vi "R45_2-RT.vi"() -> ()   [LabVIEW 2016]
uses:
  Faraday cup states.ctl
  Aperture states.ctl
  GV states.ctl
  <vilib>/Platform/TimedLoop/XDataNode/timing_clust.ctl
  <vilib>/Platform/TimedLoop/XDataNode/nitl_modes.ctl
  <vilib>/Platform/TimedLoop/XDataNode/wakeup.ctl
  Glassman Control.ctl
  GP307 cluster.ctl
  <vilib>/FPGAPlugInAG/cRIO-9074/niLvFpga_Open_cRIO-9074.vi
  <vilib>/Utility/error.llb/Error Cluster From Error Code.vi
  <vilib>/rvi/errors/niLvFpgaAdjustHostInterfaceError.vi
  <vilib>/functionblocks/Control/PID/PID.vi
  <vilib>/rvi/interface/nirviOpenFPGA/nirviOpenFPGA.xnode
  Slow-Switching-Control/FPGA Bitfiles/Controlsoftware2_FPGATarget8_R45-2-FPGA_XDn2JZv1h+E.lvbitx
  R45_2-FPGA.vi
  <vilib>/Platform/TimedLoop/XDataNode/XDataNode.xnode
  <vilib>/rvi/interface/nirviReadWriteControl/nirviReadWriteControl.xnode
  <vilib>/functionblocks/FB Core/FB Core.xnode
  Gate Valve Readback.ctl
  Aperture Readback.ctl
  Faraday Cup Readback.ctl
  Glassman Readback.ctl
  <vilib>/Platform/TimedLoop/XDataNode/XDNodeRunTimeDep.lvlib
  <vilib>/functionblocks/NI_FunctionBlock Libraries.lvlib
  NiFpgaLv.dll
panel:
  out "Error Reporter":errorcluster
  in  "Tab Control":T1(tab)
  out "HV readback loop error":errorcluster
  out "R45 ExB 1 HV Enable":bool
  out "R45 ExB 1 voltage set":dbl
  out "HV control loop error":errorcluster
  out "ExB 1- I read":dbl
  out "ExB 1- V read":dbl
  out "ExB 2+ I read":dbl
  out "ExB 2+ V read":dbl
  out "ExB 2- I read":dbl
  out "ExB 2- V read":dbl
  out "X-steerer Mag I read":dbl
  out "X-steerer Mag V read":dbl
  out "R45 ExB 2 HV Enable":bool
  out "R45 ExB 2 voltage set":dbl
  out "X-Steerer Magnet current set":dbl
  out "ExB 1+ I read":dbl
  out "ExB 1+ V read":dbl
  out "GRM magnet current set":dbl
  out "GFM read string":string
  in  "proportional gain (Kc) - GFM":dbl=1.0
  in  "integral time (Ti, min) - GFM":dbl=0.01
  in  "derivative time (Td, min) - GFM":dbl
  in  "output high - GFM":dbl=205.0
  in  "output low - GFM":dbl
  out "GFM field read":u8[](array[numeric])
  out "GFM field":dbl format="%#_8f"
  out "GFM loop error":errorcluster
  out "ExB 2 PS loop error":errorcluster
  out "ExB 1 PS loop error":errorcluster
  out "GFM command":u8[](array[numeric])
  out "R45 ExB 2 command string":string
  out "R45 ExB 2 command array":u8[](array[numeric])
  out "ExB #2 magnet current set":dbl
  out "GFM command string":string
  out "GFM field set":dbl
  out "ExB #1 magnet current set":dbl
  out "R45 ExB 1 command string":string
  out "R45 ExB 1 command array":u8[](array[numeric])
  out "Vacuum readback error":errorcluster
  out "Ion Gauge 3-2":u8[](array[numeric])
  out "Convectron gauge 3-2":u8[](array[numeric])
  out "Ion gauge 2-2":u8[](array[numeric])
  out "Ion gauge 2-1":u8[](array[numeric])
  out "Convectron 3-1":u8[](array[numeric])
  out "Ion gauge 3-1":u8[](array[numeric])
  out "Convectron 2-2":u8[](array[numeric])
  out "Convectron 2-1":u8[](array[numeric])
  out "Ion Gauge 4-1":u8[](array[numeric])
  out "Convectron Gauge 4-1":u8[](array[numeric])
  out "Ion Gauge 4-2":u8[](array[numeric])
  out "Convectron Gauge 4-2":u8[](array[numeric])
  out "R45 Quad  vac gauge cluster":T2
  out "R45 Detector vac gauge cluster":T2
  out "R45 ExB Slot vac gauge cluster":T2
  out "Vac cluster 2 Ion Guage Interlock":bool
  out "Vac cluster 3 Ion Guage Interlock":bool
  out "Vac cluster 4 Ion Guage Interlock":bool
  out "Interlock readbacks Loop error":errorcluster
  out "Vac cluster 1 Gauge Interlock":bool
  out "Vac cluster 1 Interlock bypass":bool
  out "Switch Object Vac Interlock":bool
  out "Switch Object Interlock Bypass":bool
  out "Vac cluster 2 Interlock bypass":bool
  out "Vac cluster 4 Interlock bypass":bool
  out "Vac cluster 3 Interlock bypass":bool
  out "Turbo 2 GV Status":T3
  out "Turbo 1 GV Status":T3
  out "Beamline GV 3 Status":T3
  out "Beamline GV 2 Status":T3
  out "R45 Switching Mag GV Status":T3
  out "Turbo 3 GV Status":T3
  out "Detector FC status":T4
  out "Detector Aperture status":T5
  out "Detector Aperture Position":cluster{"IN sensor":bool, "OUT sensor":bool}
  out "Turbo 3 GV Status":T6
  out "Turbo 2 GV Status":T6
  out "Beamline GV 3 Status":T6
  out "Turbo 1 GV Status":T6
  out "R45 Switching Mag GV Status":T6
  out "ExB Slot Aperture Position":cluster{"IN sensor":bool, "OUT sensor":bool}
  out "Detector FC Position":cluster{"IN sensor":bool, "OUT sensor":bool}
  out "Beamline GV 2 Status":T6
  out "ExB Slot Aperture Status":T5
  out "Actuator loop error":errorcluster
  out "R45 Detector FC insert":bool
  out "R45 Detector Aperture insert":bool
  out "R45 ExB Slot Aperture insert":bool
  out "R45 Turbo 3 GV":bool
  out "R45 Turbo 2 GV":bool
  out "R45 Switching Magnet GV":bool
  out "R45 Turbo 1 GV":bool
  out "R45 Beamline GV 3":bool
  out "R45 Beamline GV 2":bool
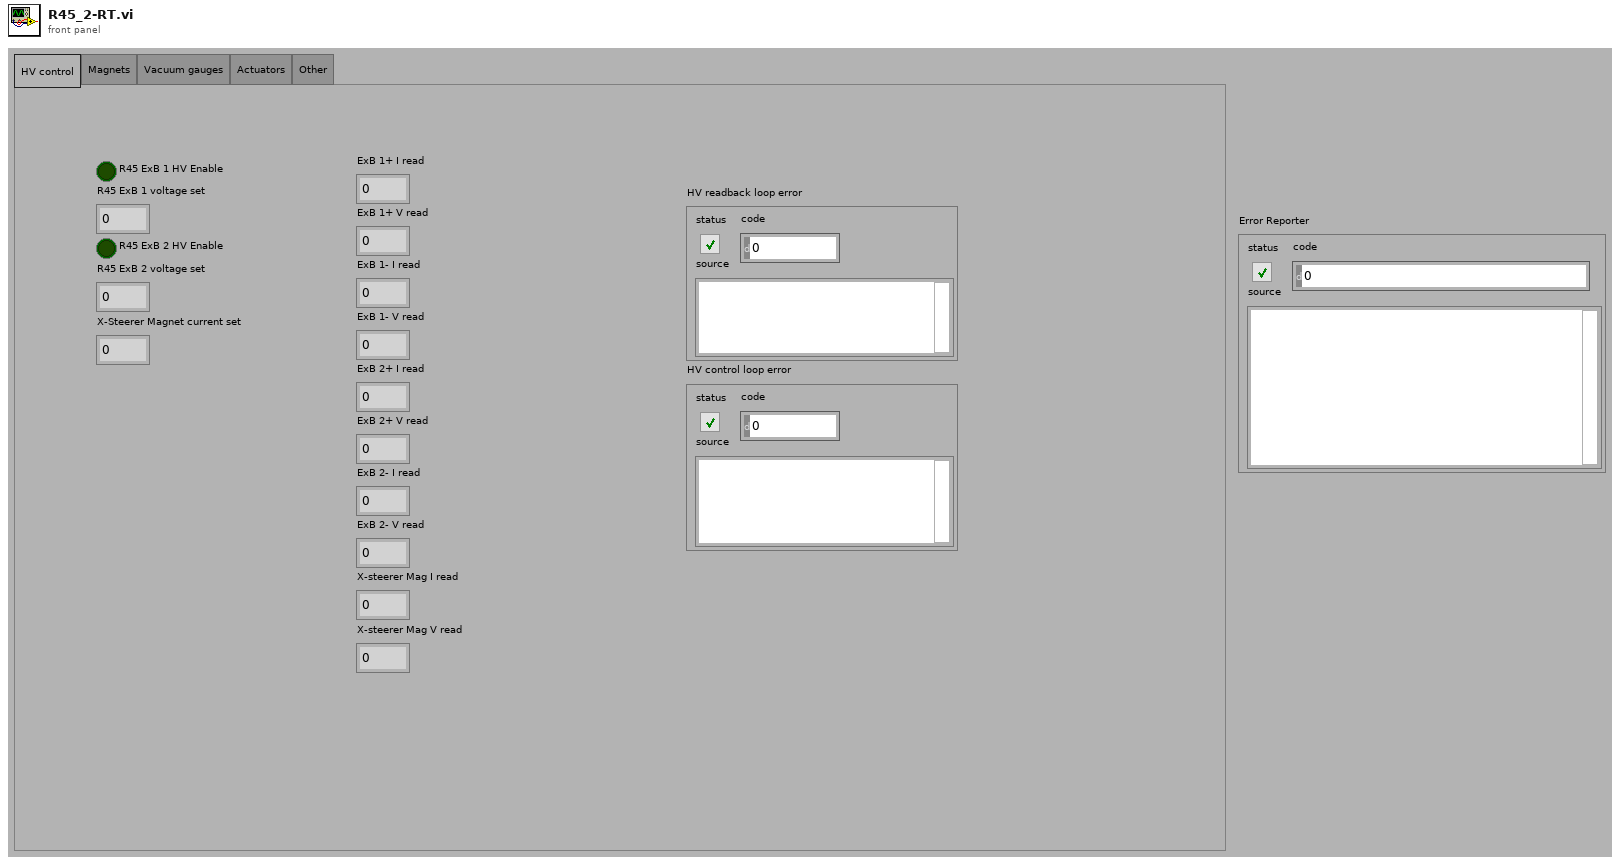
[diagram p1: front panel]
types:
  T1 = enum32{"HV control", "Magnets", "Vacuum gauges", "Actuators", "Other"}
  T2 = cluster{"Ion gauge 1":string, "Convectron  Gauge 1 ":string, "Ion Gauge 2":string, "Convectrom Gauge 2":string}
  T3 = typedef "GV states.ctl" = enum16{"status unclear", "closed", "open"}
  T4 = typedef "Faraday cup states.ctl" = enum16{"FC status unclear", "FC in", "FC out"}
  T5 = typedef "Aperture states.ctl" = enum16{"Aperture status unclear", "Aperture in", "Aperture out"}
  T6 = cluster{"OPEN sensor":bool, "Closed sensor":bool}
  T7 = typedef "XDNodeRunTimeDep.lvlib/timing_clust.ctl" = cluster{"Expected End [f-1]":u64, "Actual End [f-1]":u64, "Finished Late? [f-1]":bool, "Expected End [i-1]":u64, "Actual End [i-1]":u64, "Finished Late? [i-1]":bool, "Expected Start [i]":u64, "Actual Start [i]":u64, "Expected Start [f]":u64, "Actual Start [f]":u64, "Source Name":string, "Structure Name":string, "Period":i64, "Deadline":i64, "Offset":i64, "Start":i64, "Priority":i32, "Timeout":i32, "Mode":T8, "Wakeup Reason":T9, "Error":errorcluster, "Source Type":string, "Secondary Source Type":string, "Global End Time":u64, "Global Start Time":u64, "Frame Duration":u64, "Iteration Duration":u64, "Assigned CPU":i32, "I/O Scan Engine Mode":u32}
  T8 = typedef "XDNodeRunTimeDep.lvlib/nitl_modes.ctl" = enum32{"No Change", "Process missed periods, maintain original phase", "Discard missed periods, maintain original phase", "Process missed periods, ignore original phase", "Discard missed periods, ignore original phase"}
  T9 = typedef "XDNodeRunTimeDep.lvlib/wakeup.ctl" = enum32{"Normal", "Aborted", "Asynchronous wakeup", "Timing source error", "Timed loop error", "Timeout"}
  T10 = typedef "GP307 cluster.ctl" = cluster{"Ion gauge 1":string, "Convectron  Gauge 1 ":string, "Ion Gauge 2":string, "Convectrom Gauge 2":string}
  T11 = typedef "Glassman Control.ctl" = cluster{"V-program":fxp<+/-,20,5>, "HV Enable":bool}
  T12 = typedef "Gate Valve Readback.ctl" = cluster{"OPEN sensor":bool, "Closed sensor":bool}
  T13 = typedef "Aperture Readback.ctl" = cluster{"IN sensor":bool, "OUT sensor":bool}
  T14 = typedef "Faraday Cup Readback.ctl" = cluster{"IN sensor":bool, "OUT sensor":bool}
  T15 = typedef "Glassman Readback.ctl" = cluster{"I-monitor":fxp<+/-,26,5>, "V-monitor":fxp<+/-,26,7>}
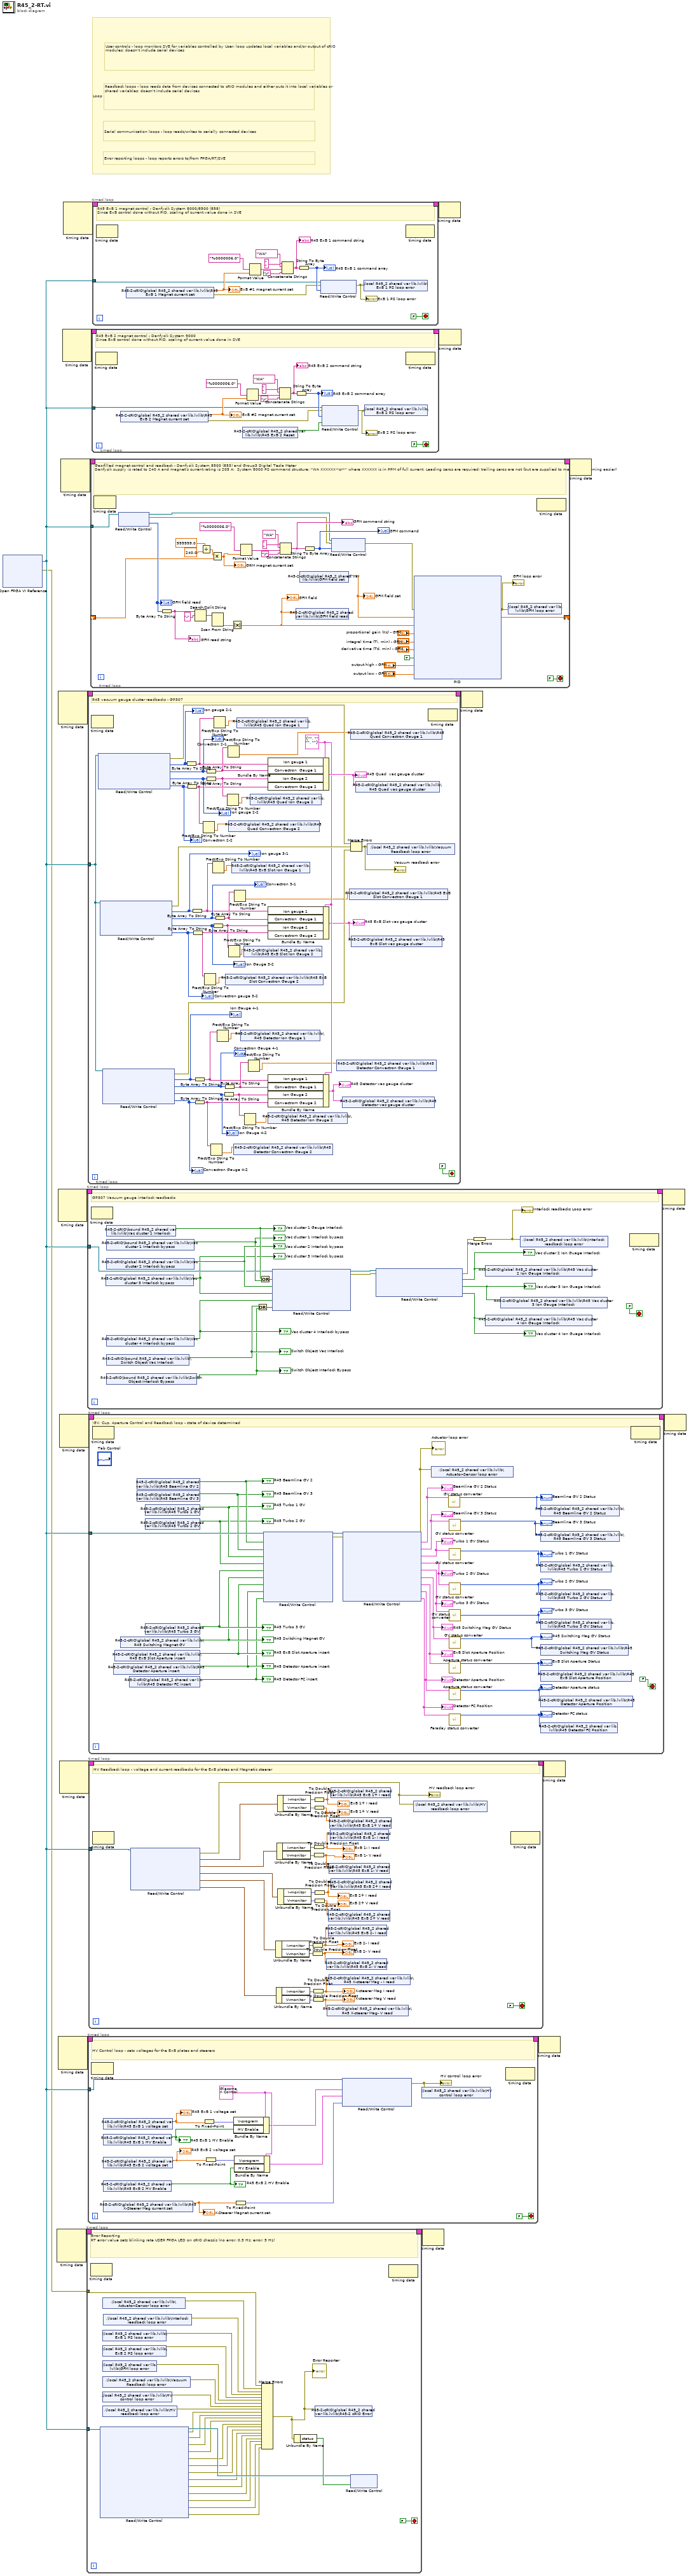
[diagram p0: block diagram]
diagram:
  # "Error reporting loops - loop reports errors to/from FPGA/RT/SVE"
  # "Serial communication loops - loop reads/writes to serially connected devices"
  # "Readback loops - loop reads data from devices connected to cRIO modules and either puts it into local variables or shared variables; doesn't include serial devices"
  # "User controls - loop monitors SVE for variables controlled by User; loop updates local variables and/or output of cRIO modules; doesn't include serial devices"
  # "Loop legend - loops are color coded by responsibility"
  n1 = xnode "Open FPGA VI Reference"() -> ("FPGA VI Reference Out"=w2:refnum<k20>, "error out"=w1:errorcluster)  [unwired: 2 in]
  n2 = node-c288() -> (w8:T7)  [unwired: 4 in]
  n3 = node-c288() -> (w16:T7)  [unwired: 4 in]
  n4 = node-c288() -> (w18:T7)  [unwired: 4 in]
  n5 = node-c288() -> (w6:T7)  [unwired: 4 in]
  n6 = node-c288() -> (w14:T7)  [unwired: 4 in]
  n7 = node-c288() -> (w4:T7)  [unwired: 4 in]
  n8 = node-c288() -> (w20:T7)  [unwired: 4 in]
  n9 = node-c288() -> (w12:T7)  [unwired: 4 in]
  n10 = node-c288() -> (w10:T7)  [unwired: 4 in]
  n11 = timed-loop {
    timing: w8 -> [_]
    timing-out: [_] -> w7
    tunnel: w2 -> [w39]
    tunnel: w1 -> [w23]
    stop <- FALSE stop-if-true
    # "Error Reporting\nRT error value sets blinking rate USER FPGA LED on cRIO chassis (no error: 0.5 Hz; error: 5 Hz)"
    n12 = node-c288() -> ()  [unwired: 1 in, 1 out]
    n13 = xnode "Read/Write Control"("FPGA VI Reference In"=w39) -> ("FPGA VI Reference Out"=w38:refnum<k20>, "error out"=w37:errorcluster, "ExB 1 PS error"=w36:errorcluster, "ExB 2 PS error"=w35:errorcluster, "GFM ps error"=w34:errorcluster, "GFM Hall Probe error"=w33:errorcluster, "HV Readback Loop"=w32:errorcluster, "HV Control Loop error"=w31:errorcluster, "Vacuum Gauge 2 error"=w30:errorcluster, "Vacuum Gauge 3 error"=w29:errorcluster, "Vacuum Gauge 4 error"=w28:errorcluster, "Vac and GV  interlock error"=w24:errorcluster, "Position-Status Sensor error"=w25:errorcluster, "Cup-Aperture Control Loop Error"=w26:errorcluster)  [unwired: 1 in]
    n14 = shared-variable ".\\local R45_2 shared var lib.lvlib\\Actuator-Sensor loop error"() -> (w21:errorcluster)  [unwired: 1 in, 1 out]
    n15 = shared-variable ".\\local R45_2 shared var lib.lvlib\\ExB 1 PS loop error"() -> (w45:errorcluster)  [unwired: 1 in, 1 out]
    n16 = shared-variable ".\\local R45_2 shared var lib.lvlib\\ExB 2 PS loop error"() -> (w44:errorcluster)  [unwired: 1 in, 1 out]
    n17 = shared-variable ".\\local R45_2 shared var lib.lvlib\\GFM loop error"() -> (w43:errorcluster)  [unwired: 1 in, 1 out]
    n18 = shared-variable ".\\local R45_2 shared var lib.lvlib\\Vacuum Readback loop error"() -> (w42:errorcluster)  [unwired: 1 in, 1 out]
    n19 = shared-variable ".\\local R45_2 shared var lib.lvlib\\HV control loop error"() -> (w41:errorcluster)  [unwired: 1 in, 1 out]
    n20 = shared-variable ".\\local R45_2 shared var lib.lvlib\\HV readback loop error"() -> (w40:errorcluster)  [unwired: 1 in, 1 out]
    n21 = shared-variable ".\\local R45_2 shared var lib.lvlib\\Interlock readback loop error"() -> (w22:errorcluster)  [unwired: 1 in, 1 out]
    n22 = Merge Errors(w23, w21, w22, w45, w44, w43, w42, w41, w40, w37, w36, w35, w34, w33, w32, w31, w30, w29, w28, w24, w25, w26) -> (w47:errorcluster)
    "Error Reporter" <- w47
    n23 = Unbundle By Name(w47) -> ("status"=w46:bool)
    n24 = shared-variable "R45-2-cRIO\\global R45_2 shared var lib.lvlib\\R45-2 cRIO Error"(w47) -> ()  [unwired: 1 in, 1 out]
    n25 = xnode "Read/Write Control"("FPGA VI Reference In"=w38, "RT error"=w46) -> ()  [unwired: 1 in, 2 out]
    n26 = node-c288() -> ()  [unwired: 1 in, 1 out]
  }
  n27 = timed-loop {
    tunnel: w2 -> [w55]
    timing: w16 -> [_]
    timing-out: [_] -> w15
    stop <- FALSE stop-if-true
    # "GP307 Vacuum gauge interlock readbacks"
    n28 = node-c288() -> ()  [unwired: 1 in, 1 out]
    n29 = shared-variable "R45-2-cRIO\\global R45_2 shared var lib.lvlib\\Vac cluster 3 Interlock bypass"() -> (w50:bool)  [unwired: 1 in, 1 out]
    "Vac cluster 3 Interlock bypass" <- w50
    n30 = shared-variable "R45-2-cRIO\\bound R45_2 shared var lib.lvlib\\Vac cluster 1 Interlock"() -> (w59:bool)  [unwired: 1 in, 1 out]
    "Vac cluster 1 Gauge Interlock" <- w59
    n31 = shared-variable "R45-2-cRIO\\bound R45_2 shared var lib.lvlib\\Vac cluster 1 Interlock bypass"() -> (w51:bool)  [unwired: 1 in, 1 out]
    "Vac cluster 1 Interlock bypass" <- w51
    n32 = shared-variable "R45-2-cRIO\\global R45_2 shared var lib.lvlib\\Vac cluster 2 Interlock bypass"() -> (w56:bool)  [unwired: 1 in, 1 out]
    "Vac cluster 2 Interlock bypass" <- w56
    n33 = shared-variable "R45-2-cRIO\\global R45_2 shared var lib.lvlib\\Vac cluster 4 Interlock bypass"() -> (w57:bool)  [unwired: 1 in, 1 out]
    "Vac cluster 4 Interlock bypass" <- w57
    n34 = shared-variable "R45-2-cRIO\\bound R45_2 shared var lib.lvlib\\Switch Object Vac Interlock"() -> (w58:bool)  [unwired: 1 in, 1 out]
    "Switch Object Vac Interlock" <- w58
    n35 = shared-variable "R45-2-cRIO\\bound R45_2 shared var lib.lvlib\\Switch Object Interlock Bypass"() -> (w53:bool)  [unwired: 1 in, 1 out]
    "Switch Object Interlock Bypass" <- w53
    n36 = Or(x=w58, y=w53) -> (x .or. y?=w54:bool)
    n37 = Or(x=w59, y=w51) -> (x .or. y?=w52:bool)
    n38 = xnode "Read/Write Control"("FPGA VI Reference In"=w55, "Vac cluster 1 Gauge Interlock"=w52, "Vac cluster 2 Interlock bypass"=w56, "Vac cluster 3 Interlock bypass"=w50, "Vac cluster 4 Interlock bypass"=w57, "Switch Object Interlock"=w54) -> ("FPGA VI Reference Out"=w61:refnum<k20>, "error out"=w60:errorcluster)  [unwired: 1 in]
    n39 = xnode "Read/Write Control"("FPGA VI Reference In"=w61, "error in"=w60) -> ("error out"=w63:errorcluster, "Vac cluster 2 Ion Gauge Interlock"=w64:bool, "Vac cluster 3 Ion Gauge Interlock"=w66:bool, "Vac cluster 4 Ion Gauge Interlock"=w65:bool)  [unwired: 1 out]
    "Vac cluster 2 Ion Guage Interlock" <- w64
    "Vac cluster 3 Ion Guage Interlock" <- w66
    "Vac cluster 4 Ion Guage Interlock" <- w65
    n40 = Merge Errors(w63) -> (w62:errorcluster)
    "Interlock readbacks Loop error" <- w62
    n41 = shared-variable "R45-2-cRIO\\global R45_2 shared var lib.lvlib\\R45 Vac cluster 2 Ion Gauge Interlock"(w64) -> ()  [unwired: 1 in, 1 out]
    n42 = shared-variable "R45-2-cRIO\\global R45_2 shared var lib.lvlib\\R45 Vac cluster 4 Ion Gauge Interlock"(w65) -> ()  [unwired: 1 in, 1 out]
    n43 = shared-variable "R45-2-cRIO\\global R45_2 shared var lib.lvlib\\R45 Vac cluster 3 Ion Gauge Interlock"(w66) -> ()  [unwired: 1 in, 1 out]
    n44 = shared-variable ".\\local R45_2 shared var lib.lvlib\\Interlock readback loop error"(w62) -> ()  [unwired: 1 in, 1 out]
    n45 = node-c288() -> ()  [unwired: 1 in, 1 out]
  }
  n46 = timed-loop {
    tunnel: w2 -> [w93]
    timing: w18 -> [_]
    timing-out: [_] -> w17
    stop <- FALSE stop-if-true
    w104 = T10 {"Ion gauge 1"="", "Convectron  Gauge 1 "="", "Ion Gauge 2"="", "Convectrom Gauge 2"=""} ("Ion gauge cluster control")
    # "R45 vacuum gauge cluster readbacks - GP307"
    n47 = node-c288() -> ()  [unwired: 1 in, 1 out]
    n48 = xnode "Read/Write Control"("FPGA VI Reference In"=w93) -> ("error out"=w83:errorcluster, "Vac Cluster 2 Ion Gauge 1"=w92:u8[], "Vac Cluster 2 Convectron 1"=w91:u8[], "Vac Cluster 2 Ion Gauge 2"=w90:u8[], "Vac Cluster 2 Convectron 2"=w89:u8[])  [unwired: 1 in, 1 out]
    "Ion gauge 2-1" <- w92
    "Convectron 2-1" <- w91
    "Ion gauge 2-2" <- w90
    "Convectron 2-2" <- w89
    n49 = xnode "Read/Write Control"("FPGA VI Reference In"=w93) -> ("error out"=w115:errorcluster, "Vac Cluster 3 Ion Gauge 1"=w113:u8[], "Vac Cluster 3 Convectron 1"=w112:u8[], "Vac Cluster 3 Convectron 2"=w110:u8[], "Vac Cluster 3 Convectron 2"=w111:u8[])  [unwired: 1 in, 1 out]
    "Ion gauge 3-1" <- w113
    "Convectron 3-1" <- w112
    "Convectron gauge 3-2" <- w111
    "Ion Gauge 3-2" <- w110
    n50 = xnode "Read/Write Control"("FPGA VI Reference In"=w93) -> ("error out"=w82:errorcluster, "Vac Cluster 4 Ion Gauge 1"=w96:u8[], "Vac Cluster 4 Convectron 1"=w98:u8[], "Vac Cluster 4 Ion Gauge 2"=w99:u8[], "Vac Cluster 4 Convectron 2"=w97:u8[])  [unwired: 1 in, 1 out]
    "Ion Gauge 4-1" <- w96
    "Convectron Gauge 4-1" <- w98
    "Ion Gauge 4-2" <- w99
    "Convectron Gauge 4-2" <- w97
    n51 = Byte Array To String(unsigned byte array=w92) -> (string=w108:string)
    n52 = Byte Array To String(unsigned byte array=w89) -> (string=w86:string)
    n53 = Byte Array To String(unsigned byte array=w113) -> (string=w107:string)
    n54 = Byte Array To String(unsigned byte array=w111) -> (string=w88:string)
    n55 = Byte Array To String(unsigned byte array=w96) -> (string=w100:string)
    n56 = Byte Array To String(unsigned byte array=w97) -> (string=w94:string)
    n57 = Fract/Exp String To Number(string=w86) -> (number=w71:dbl)  [unwired: 3 in, 1 out]
    n58 = Fract/Exp String To Number(string=w88) -> (number=w75:dbl)  [unwired: 3 in, 1 out]
    n59 = Byte Array To String(unsigned byte array=w91) -> (string=w105:string)
    n60 = Byte Array To String(unsigned byte array=w90) -> (string=w85:string)
    n61 = Fract/Exp String To Number(string=w94) -> (number=w78:dbl)  [unwired: 3 in, 1 out]
    n62 = Fract/Exp String To Number(string=w107) -> (number=w77:dbl)  [unwired: 3 in, 1 out]
    n63 = Byte Array To String(unsigned byte array=w110) -> (string=w87:string)
    n64 = Fract/Exp String To Number(string=w108) -> (number=w73:dbl)  [unwired: 3 in, 1 out]
    n65 = Byte Array To String(unsigned byte array=w112) -> (string=w106:string)
    n66 = Fract/Exp String To Number(string=w100) -> (number=w81:dbl)  [unwired: 3 in, 1 out]
    n67 = Byte Array To String(unsigned byte array=w99) -> (string=w95:string)
    n68 = Byte Array To String(unsigned byte array=w98) -> (string=w101:string)
    n69 = shared-variable "R45-2-cRIO\\global R45_2 shared var lib.lvlib\\R45 ExB Slot Convectron Gauge 2"(w75) -> ()  [unwired: 1 in, 1 out]
    n70 = Fract/Exp String To Number(string=w85) -> (number=w72:dbl)  [unwired: 3 in, 1 out]
    n71 = Fract/Exp String To Number(string=w105) -> (number=w70:dbl)  [unwired: 3 in, 1 out]
    n72 = shared-variable "R45-2-cRIO\\global R45_2 shared var lib.lvlib\\R45 Quad Convectron Gauge 2"(w71) -> ()  [unwired: 1 in, 1 out]
    n73 = Fract/Exp String To Number(string=w87) -> (number=w76:dbl)  [unwired: 3 in, 1 out]
    n74 = shared-variable "R45-2-cRIO\\global R45_2 shared var lib.lvlib\\R45 ExB Slot Ion Gauge 1"(w77) -> ()  [unwired: 1 in, 1 out]
    n75 = shared-variable "R45-2-cRIO\\global R45_2 shared var lib.lvlib\\R45 Detector Convectron Gauge 2"(w78) -> ()  [unwired: 1 in, 1 out]
    n76 = Fract/Exp String To Number(string=w106) -> (number=w74:dbl)  [unwired: 3 in, 1 out]
    n77 = shared-variable "R45-2-cRIO\\global R45_2 shared var lib.lvlib\\R45 Quad Ion Gauge 1"(w73) -> ()  [unwired: 1 in, 1 out]
    n78 = shared-variable "R45-2-cRIO\\global R45_2 shared var lib.lvlib\\R45 Detector Ion Gauge 1"(w81) -> ()  [unwired: 1 in, 1 out]
    n79 = shared-variable "R45-2-cRIO\\global R45_2 shared var lib.lvlib\\R45 ExB Slot Ion Gauge 2"(w76) -> ()  [unwired: 1 in, 1 out]
    n80 = Fract/Exp String To Number(string=w95) -> (number=w80:dbl)  [unwired: 3 in, 1 out]
    n81 = Fract/Exp String To Number(string=w101) -> (number=w79:dbl)  [unwired: 3 in, 1 out]
    n82 = shared-variable "R45-2-cRIO\\global R45_2 shared var lib.lvlib\\R45 Quad Ion Gauge 2"(w72) -> ()  [unwired: 1 in, 1 out]
    n83 = shared-variable "R45-2-cRIO\\global R45_2 shared var lib.lvlib\\R45 Detector Ion Gauge 2"(w80) -> ()  [unwired: 1 in, 1 out]
    n84 = Bundle By Name(cluster=w104, "Ion gauge 1"=w108, "Convectron  Gauge 1"=w105, "Ion Gauge 2"=w85, "Convectrom Gauge 2"=w86) -> (w109:T10)
    "R45 Quad  vac gauge cluster" <- w109
    n85 = Bundle By Name(cluster=w104, "Ion gauge 1"=w107, "Convectron  Gauge 1"=w106, "Ion Gauge 2"=w88, "Convectrom Gauge 2"=w87) -> (w102:T10)
    "R45 ExB Slot vac gauge cluster" <- w102
    n86 = Bundle By Name(cluster=w104, "Ion gauge 1"=w100, "Convectron  Gauge 1"=w101, "Ion Gauge 2"=w95, "Convectrom Gauge 2"=w94) -> (w103:T10)
    "R45 Detector vac gauge cluster" <- w103
    n87 = shared-variable "R45-2-cRIO\\global R45_2 shared var lib.lvlib\\R45 Detector Convectron Gauge 1"(w79) -> ()  [unwired: 1 in, 1 out]
    n88 = shared-variable "R45-2-cRIO\\global R45_2 shared var lib.lvlib\\R45 Detector vac gauge cluster"(w103) -> ()  [unwired: 1 in, 1 out]
    n89 = shared-variable "R45-2-cRIO\\global R45_2 shared var lib.lvlib\\R45 ExB Slot Convectron Gauge 1"(w74) -> ()  [unwired: 1 in, 1 out]
    n90 = shared-variable "R45-2-cRIO\\global R45_2 shared var lib.lvlib\\R45 Quad Convectron Gauge 1"(w70) -> ()  [unwired: 1 in, 1 out]
    n91 = Merge Errors(w83, w115, w82) -> (w84:errorcluster)
    "Vacuum readback error" <- w84
    n92 = shared-variable "R45-2-cRIO\\global R45_2 shared var lib.lvlib\\R45 ExB Slot vac gauge cluster"(w102) -> ()  [unwired: 1 in, 1 out]
    n93 = shared-variable "R45-2-cRIO\\global R45_2 shared var lib.lvlib\\R45 Quad vac gauge cluster"(w109) -> ()  [unwired: 1 in, 1 out]
    n94 = shared-variable ".\\local R45_2 shared var lib.lvlib\\Vacuum Readback loop error"(w84) -> ()  [unwired: 1 in, 1 out]
    n95 = node-c288() -> ()  [unwired: 1 in, 1 out]
  }
  n96 = timed-loop {
    timing: w6 -> [_]
    timing-out: [_] -> w5
    tunnel: w2 -> [w131]
    stop <- FALSE stop-if-true
    w127 = T11 {"V-program"=0.0, "HV Enable"=FALSE} ("Glassman Control")
    # "HV Control loop - sets voltages for the ExB plates and steerers"
    n97 = node-c288() -> ()  [unwired: 1 in, 1 out]
    n98 = shared-variable "R45-2-cRIO\\global R45_2 shared var lib.lvlib\\R45 ExB 1 voltage set"() -> (w124:dbl)  [unwired: 1 in, 1 out]
    "R45 ExB 1 voltage set" <- w124
    n99 = shared-variable "R45-2-cRIO\\global R45_2 shared var lib.lvlib\\R45 ExB 1 HV Enable"() -> (w125:bool)  [unwired: 1 in, 1 out]
    "R45 ExB 1 HV Enable" <- w125
    n100 = shared-variable "R45-2-cRIO\\global R45_2 shared var lib.lvlib\\R45 ExB 2 voltage set"() -> (w122:dbl)  [unwired: 1 in, 1 out]
    "R45 ExB 2 voltage set" <- w122
    n101 = shared-variable "R45-2-cRIO\\global R45_2 shared var lib.lvlib\\R45 ExB 2 HV Enable"() -> (w120:bool)  [unwired: 1 in, 1 out]
    "R45 ExB 2 HV Enable" <- w120
    n102 = shared-variable "R45-2-cRIO\\global R45_2 shared var lib.lvlib\\R45 X-Steerer Mag current set"() -> (w130:dbl)  [unwired: 1 in, 1 out]
    "X-Steerer Magnet current set" <- w130
    n103 = To Fixed-Point(number=w124) -> (fixed-point=w123:fxp<+/-,20,5>)  [unwired: 1 in]
    n104 = To Fixed-Point(number=w122) -> (fixed-point=w121:fxp<+/-,20,5>)  [unwired: 1 in]
    n105 = Bundle By Name(cluster=w127, "V-program"=w123, "HV Enable"=w125) -> (w126:T11)
    n106 = Bundle By Name(cluster=w127, "V-program"=w121, "HV Enable"=w120) -> (w128:T11)
    n107 = To Fixed-Point(number=w130) -> (fixed-point=w129:fxp<+/-,20,5>)  [unwired: 1 in]
    n108 = xnode "Read/Write Control"("FPGA VI Reference In"=w131, "ExB 1 - Voltage Set"=w126, "ExB 2 - Voltage Set"=w128, "Mag Steerer I-program"=w129) -> ("error out"=w119:errorcluster)  [unwired: 1 in, 1 out]
    "HV control loop error" <- w119
    n109 = shared-variable ".\\local R45_2 shared var lib.lvlib\\HV control loop error"(w119) -> ()  [unwired: 1 in, 1 out]
    n110 = node-c288() -> ()  [unwired: 1 in, 1 out]
  }
  n111 = timed-loop {
    tunnel: w2 -> [w164]
    timing: w14 -> [_]
    timing-out: [_] -> w13
    stop <- FALSE stop-if-true
    # "GV, Cup, Aperture Control and Readback loop - state of device determined"
    n112 = node-c288() -> ()  [unwired: 1 in, 1 out]
    n113 = shared-variable "R45-2-cRIO\\global R45_2 shared var lib.lvlib\\R45 Detector Aperture insert"() -> (w154:bool)  [unwired: 1 in, 1 out]
    "R45 Detector Aperture insert" <- w154
    n114 = shared-variable "R45-2-cRIO\\global R45_2 shared var lib.lvlib\\R45 ExB Slot Aperture insert"() -> (w155:bool)  [unwired: 1 in, 1 out]
    "R45 ExB Slot Aperture insert" <- w155
    n115 = shared-variable "R45-2-cRIO\\global R45_2 shared var lib.lvlib\\R45 Switching Magnet GV"() -> (w156:bool)  [unwired: 1 in, 1 out]
    "R45 Switching Magnet GV" <- w156
    n116 = shared-variable "R45-2-cRIO\\global R45_2 shared var lib.lvlib\\R45 Detector FC insert"() -> (w153:bool)  [unwired: 1 in, 1 out]
    "R45 Detector FC insert" <- w153
    n117 = shared-variable "R45-2-cRIO\\global R45_2 shared var lib.lvlib\\R45 Beamline GV 2"() -> (w161:bool)  [unwired: 1 in, 1 out]
    "R45 Beamline GV 2" <- w161
    n118 = shared-variable "R45-2-cRIO\\global R45_2 shared var lib.lvlib\\R45 Beamline GV 3"() -> (w160:bool)  [unwired: 1 in, 1 out]
    "R45 Beamline GV 3" <- w160
    n119 = shared-variable "R45-2-cRIO\\global R45_2 shared var lib.lvlib\\R45 Turbo 1 GV"() -> (w159:bool)  [unwired: 1 in, 1 out]
    "R45 Turbo 1 GV" <- w159
    n120 = shared-variable "R45-2-cRIO\\global R45_2 shared var lib.lvlib\\R45 Turbo 2 GV"() -> (w158:bool)  [unwired: 1 in, 1 out]
    "R45 Turbo 2 GV" <- w158
    n121 = shared-variable "R45-2-cRIO\\global R45_2 shared var lib.lvlib\\R45 Turbo 3 GV"() -> (w157:bool)  [unwired: 1 in, 1 out]
    "R45 Turbo 3 GV" <- w157
    n122 = xnode "Read/Write Control"("FPGA VI Reference In"=w164, "Beamline GV 2"=w161, "Beamline GV 3"=w160, "Turbo 1 GV"=w159, "Turbo 2 GV"=w158, "Turbo 3 GV"=w157, "Switching Magnet GV"=w156, "ExB Slot Aperture insert"=w155, "Detector Aperture insert"=w154, "Detector FC insert"=w153) -> ("FPGA VI Reference Out"=w163:refnum<k20>, "error out"=w162:errorcluster)  [unwired: 1 in]
    n123 = xnode "Read/Write Control"("FPGA VI Reference In"=w163, "error in"=w162) -> ("error out"=w152:errorcluster, "Beamline GV 2 Status"=w140:T12, "Beamline GV 3 Status"=w141:T12, "Turbo 1 GV Status"=w139:T12, "Turbo 2 GV Status"=w142:T12, "Turbo 3 GV Status"=w143:T12, "R45 Switching Mag GV Status"=w145:T12, "ExB Slot Aperture Position"=w147:T13, "Detector Aperture Position"=w149:T13, "Detector FC Position"=w151:T14)  [unwired: 1 out]
    "Beamline GV 2 Status" <- w140
    "Beamline GV 3 Status" <- w141
    "Turbo 1 GV Status" <- w139
    "Turbo 2 GV Status" <- w142
    "Turbo 3 GV Status" <- w143
    "R45 Switching Mag GV Status" <- w145
    "ExB Slot Aperture Position" <- w147
    "Detector Aperture Position" <- w149
    "Detector FC Position" <- w151
    "Actuator loop error" <- w152
    n124 = shared-variable ".\\local R45_2 shared var lib.lvlib\\Actuator-Sensor loop error"(w152) -> ()  [unwired: 1 in, 1 out]
    n125 = call "GV status converter.vi"("Gate Valve"=w140) -> ("GV Status"=w138:T3)  [unwired: 10 in]
    "Beamline GV 2 Status" <- w138
    n126 = call "GV status converter.vi"("Gate Valve"=w141) -> ("GV Status"=w137:T3)  [unwired: 10 in]
    "Beamline GV 3 Status" <- w137
    n127 = call "GV status converter.vi"("Gate Valve"=w139) -> ("GV Status"=w136:T3)  [unwired: 10 in]
    "Turbo 1 GV Status" <- w136
    n128 = call "GV status converter.vi"("Gate Valve"=w142) -> ("GV Status"=w135:T3)  [unwired: 10 in]
    "Turbo 2 GV Status" <- w135
    n129 = call "GV status converter.vi"("Gate Valve"=w143) -> ("GV Status"=w134:T3)  [unwired: 10 in]
    "Turbo 3 GV Status" <- w134
    n130 = call "GV status converter.vi"("Gate Valve"=w145) -> ("GV Status"=w144:T3)  [unwired: 10 in]
    "R45 Switching Mag GV Status" <- w144
    n131 = call "Aperture status converter.vi"("Aperture Position"=w147) -> ("Aperture Status"=w146:T5)  [unwired: 10 in]
    "ExB Slot Aperture Status" <- w146
    n132 = call "Aperture status converter.vi"("Aperture Position"=w149) -> ("Aperture Status"=w148:T5)  [unwired: 10 in]
    "Detector Aperture status" <- w148
    n133 = call "Faraday status converter.vi"("FC Position"=w151) -> ("FC Status"=w150:T4)  [unwired: 10 in]
    "Detector FC status" <- w150
    n134 = shared-variable "R45-2-cRIO\\global R45_2 shared var lib.lvlib\\R45 Beamline GV 2 Status"(w138) -> ()  [unwired: 1 in, 1 out]
    n135 = shared-variable "R45-2-cRIO\\global R45_2 shared var lib.lvlib\\R45 Beamline GV 3 Status"(w137) -> ()  [unwired: 1 in, 1 out]
    n136 = shared-variable "R45-2-cRIO\\global R45_2 shared var lib.lvlib\\R45 Turbo 1 GV Status"(w136) -> ()  [unwired: 1 in, 1 out]
    n137 = shared-variable "R45-2-cRIO\\global R45_2 shared var lib.lvlib\\R45 Turbo 2 GV Status"(w135) -> ()  [unwired: 1 in, 1 out]
    n138 = shared-variable "R45-2-cRIO\\global R45_2 shared var lib.lvlib\\R45 Turbo 3 GV Status"(w134) -> ()  [unwired: 1 in, 1 out]
    n139 = shared-variable "R45-2-cRIO\\global R45_2 shared var lib.lvlib\\R45 Switching Mag GV Status"(w144) -> ()  [unwired: 1 in, 1 out]
    n140 = shared-variable "R45-2-cRIO\\global R45_2 shared var lib.lvlib\\R45 ExB Slot Aperture Position"(w146) -> ()  [unwired: 1 in, 1 out]
    n141 = shared-variable "R45-2-cRIO\\global R45_2 shared var lib.lvlib\\R45 Detector Aperture Position"(w148) -> ()  [unwired: 1 in, 1 out]
    n142 = shared-variable "R45-2-cRIO\\global R45_2 shared var lib.lvlib\\R45 Detector FC Position"(w150) -> ()  [unwired: 1 in, 1 out]
    n143 = node-c288() -> ()  [unwired: 1 in, 1 out]
  }
  n144 = timed-loop {
    timing: w4 -> [_]
    timing-out: [_] -> w3
    tunnel: w2 -> [w195]
    stop <- FALSE stop-if-true
    # "HV Readback loop - voltage and current readbacks for the ExB plates and Magnetic steerer"
    n145 = node-c288() -> ()  [unwired: 1 in, 1 out]
    n146 = xnode "Read/Write Control"("FPGA VI Reference In"=w195) -> ("error out"=w177:errorcluster, "ExB 1+ Monitor"=w194:T15, "ExB 1- Monitor"=w193:T15, "ExB 2+ Monitor"=w192:T15, "ExB 2- Monitor"=w191:T15, "Mag Steerer - Monitor"=w190:T15)  [unwired: 1 in, 1 out]
    "HV readback loop error" <- w177
    n147 = Unbundle By Name(w191) -> ("I-monitor"=w184:fxp<+/-,26,5>, "V-monitor"=w183:fxp<+/-,26,7>)
    n148 = Unbundle By Name(w190) -> ("I-monitor"=w182:fxp<+/-,26,5>, "V-monitor"=w181:fxp<+/-,26,7>)
    n149 = Unbundle By Name(w193) -> ("I-monitor"=w188:fxp<+/-,26,5>, "V-monitor"=w187:fxp<+/-,26,7>)
    n150 = Unbundle By Name(w194) -> ("I-monitor"=w180:fxp<+/-,26,5>, "V-monitor"=w189:fxp<+/-,26,7>)
    n151 = Unbundle By Name(w192) -> ("I-monitor"=w186:fxp<+/-,26,5>, "V-monitor"=w185:fxp<+/-,26,7>)
    n152 = To Double Precision Float(number=w184) -> (double precision float=w171:dbl)
    "ExB 2- I read" <- w171
    n153 = To Double Precision Float(number=w183) -> (double precision float=w170:dbl)
    "ExB 2- V read" <- w170
    n154 = To Double Precision Float(number=w182) -> (double precision float=w169:dbl)
    "X-steerer Mag I read" <- w169
    n155 = To Double Precision Float(number=w181) -> (double precision float=w168:dbl)
    "X-steerer Mag V read" <- w168
    n156 = To Double Precision Float(number=w188) -> (double precision float=w175:dbl)
    "ExB 1- I read" <- w175
    n157 = To Double Precision Float(number=w187) -> (double precision float=w174:dbl)
    "ExB 1- V read" <- w174
    n158 = To Double Precision Float(number=w180) -> (double precision float=w178:dbl)
    "ExB 1+ I read" <- w178
    n159 = To Double Precision Float(number=w189) -> (double precision float=w179:dbl)
    "ExB 1+ V read" <- w179
    n160 = To Double Precision Float(number=w186) -> (double precision float=w173:dbl)
    "ExB 2+ I read" <- w173
    n161 = To Double Precision Float(number=w185) -> (double precision float=w172:dbl)
    "ExB 2+ V read" <- w172
    n162 = shared-variable "R45-2-cRIO\\global R45_2 shared var lib.lvlib\\R45 ExB 2- V read"(w170) -> ()  [unwired: 1 in, 1 out]
    n163 = shared-variable "R45-2-cRIO\\global R45_2 shared var lib.lvlib\\R45 X-steerer Mag- V read"(w168) -> ()  [unwired: 1 in, 1 out]
    n164 = shared-variable "R45-2-cRIO\\global R45_2 shared var lib.lvlib\\R45 ExB 2+ V read"(w172) -> ()  [unwired: 1 in, 1 out]
    n165 = shared-variable "R45-2-cRIO\\global R45_2 shared var lib.lvlib\\R45 ExB 2- I read"(w171) -> ()  [unwired: 1 in, 1 out]
    n166 = shared-variable "R45-2-cRIO\\global R45_2 shared var lib.lvlib\\R45 ExB 1- V read"(w174) -> ()  [unwired: 1 in, 1 out]
    n167 = shared-variable "R45-2-cRIO\\global R45_2 shared var lib.lvlib\\R45 X-steerer Mag - I read"(w169) -> ()  [unwired: 1 in, 1 out]
    n168 = shared-variable "R45-2-cRIO\\global R45_2 shared var lib.lvlib\\R45 ExB 1+ V read"(w179) -> ()  [unwired: 1 in, 1 out]
    n169 = shared-variable "R45-2-cRIO\\global R45_2 shared var lib.lvlib\\R45 ExB 1- I read"(w175) -> ()  [unwired: 1 in, 1 out]
    n170 = shared-variable "R45-2-cRIO\\global R45_2 shared var lib.lvlib\\R45 ExB 1+ I read"(w178) -> ()  [unwired: 1 in, 1 out]
    n171 = shared-variable "R45-2-cRIO\\global R45_2 shared var lib.lvlib\\R45 ExB 2+ I read"(w173) -> ()  [unwired: 1 in, 1 out]
    n172 = shared-variable ".\\local R45_2 shared var lib.lvlib\\HV readback loop error"(w177) -> ()  [unwired: 1 in, 1 out]
    n173 = node-c288() -> ()  [unwired: 1 in, 1 out]
  }
  n174 = timed-loop {
    tunnel: w2 -> [w220]
    timing: w20 -> [_]
    timing-out: [_] -> w19
    shift-right: [w215] -> _
    shift-left: _ -> [w209]
    stop <- FALSE stop-if-true
    # "Gas-filled magnet control and readback - Danfysik System 8500 (853) and Group3 Digital Tesla Meter\nDanfysik supply is rated to 240 A and magnet's current rating is 205 A;  System 8000 PS command structure: \"WA XXXXXX<cr>\" where XXXXXX is in PPM of full current. Leading zeros are required; trailing zeros are not (but are supplied to make programming easier)"
    n175 = node-c288() -> ()  [unwired: 1 in, 1 out]
    n176 = xnode "Read/Write Control"("FPGA VI Reference In"=w220) -> ("FPGA VI Reference Out"=w219:refnum<k20>, "error out"=w218:errorcluster, "GFM read"=w221:u8[])  [unwired: 1 in]
    "GFM field read" <- w221
    n177 = Byte Array To String(unsigned byte array=w221) -> (string=w199:string)
    "GFM read string" <- w199
    n178 = Search/Split String(string=w199, search string/char (-)="-") -> (match + rest of string=w200:string)  [unwired: 3 out]
    n179 = Divide(x=999999.0, y=240.0) -> (x/y=w205:dbl)
    n180 = Multiply(x=w205, y=w209) -> (x*y=w206:dbl)
    "GRM magnet current set" <- w206
    n181 = Scan From String(input string=w200) -> (output 1=w201:dbl)  [unwired: 3 in, 4 out]
    n182 = Absolute Value(x=w201) -> (abs(x)=w198:dbl)
    "GFM field" <- w198
    n183 = Format Value(format string="%0000006.0", value (0)=w206) -> (output string=w227:string)  [unwired: 1 out]
    n184 = Concatenate Strings("WA", " ", w227, "\r") -> (w223:string)
    "GFM command string" <- w223
    n185 = shared-variable "R45-2-cRIO\\global R45_2 shared var lib.lvlib\\GFM field read"(w198) -> ()  [unwired: 1 in, 1 out]
    n186 = shared-variable "R45-2-cRIO\\global R45_2 shared var lib.lvlib\\GFM field set"() -> (w214:dbl)  [unwired: 1 in, 1 out]
    "GFM field set" <- w214
    n187 = String To Byte Array(string=w223) -> (unsigned byte array=w222:u8[])
    "GFM command" <- w222
    n188 = xnode "Read/Write Control"("FPGA VI Reference In"=w219, "error in"=w218, "GFM ps set"=w222) -> ("error out"=w217:errorcluster)  [unwired: 1 out]
    n189 = xnode "PID"("error in"=w217, "setpoint"=w214, "process variable"=w198, "proportional gain (Kc)"="proportional gain (Kc) - GFM", "integral time (Ti, min)"="integral time (Ti, min) - GFM", "derivative time (Td, min)"="derivative time (Td, min) - GFM", "auto? (T)"=TRUE, "output high"="output high - GFM", "output low"="output low - GFM") -> ("error out"=w216:errorcluster, "output"=w215:dbl)
    "GFM loop error" <- w216
    n190 = shared-variable ".\\local R45_2 shared var lib.lvlib\\GFM loop error"(w216) -> ()  [unwired: 1 in, 1 out]
    n191 = node-c288() -> ()  [unwired: 1 in, 1 out]
  }
  n192 = timed-loop {
    timing: w12 -> [_]
    timing-out: [_] -> w11
    tunnel: w2 -> [w299]
    stop <- FALSE stop-if-true
    # "R45 ExB 2 magnet control - Danfysik System 9000\nSince ExB control done without PID, scaling of current value done in SVE"
    n193 = node-c288() -> ()  [unwired: 1 in, 1 out]
    n194 = shared-variable "R45-2-cRIO\\global R45_2 shared var lib.lvlib\\R45 ExB 2 Magnet current set"() -> (w307:dbl, error out=w301:errorcluster)  [unwired: 1 in]
    "ExB #2 magnet current set" <- w307
    n195 = shared-variable "R45-2-cRIO\\global R45_2 shared var lib.lvlib\\R45 ExB 2 Reset"() -> (w310:bool)  [unwired: 1 in, 1 out]
    n196 = Format Value(format string="%0000006.0", value (0)=w307) -> (output string=w305:string)  [unwired: 1 out]
    n197 = Concatenate Strings("WA", " ", w305, "\r") -> (w308:string)
    "R45 ExB 2 command string" <- w308
    n198 = String To Byte Array(string=w308) -> (unsigned byte array=w306:u8[])
    "R45 ExB 2 command array" <- w306
    n199 = xnode "Read/Write Control"("FPGA VI Reference In"=w299, "error in"=w301, "ExB 2 PS set"=w306, "ExB 2 Reset"=w310) -> ("error out"=w300:errorcluster)  [unwired: 1 out]
    "ExB 2 PS loop error" <- w300
    n200 = shared-variable ".\\local R45_2 shared var lib.lvlib\\ExB 2 PS loop error"(w300) -> ()  [unwired: 1 in, 1 out]
    n201 = node-c288() -> ()  [unwired: 1 in, 1 out]
  }
  n202 = timed-loop {
    timing: w10 -> [_]
    timing-out: [_] -> w9
    tunnel: w2 -> [w315]
    stop <- FALSE stop-if-true
    # "R45 ExB 1 magnet control - Danfysik System 8000/8500 (858)\nSince ExB control done without PID, scaling of current value done in SVE"
    n203 = node-c288() -> ()  [unwired: 1 in, 1 out]
    n204 = shared-variable "R45-2-cRIO\\global R45_2 shared var lib.lvlib\\R45 ExB 1 Magnet current set"() -> (w322:dbl, error out=w316:errorcluster)  [unwired: 1 in]
    "ExB #1 magnet current set" <- w322
    n205 = Format Value(format string="%0000006.0", value (0)=w322) -> (output string=w320:string)  [unwired: 1 out]
    n206 = Concatenate Strings("WA", " ", w320, "\r") -> (w323:string)
    "R45 ExB 1 command string" <- w323
    n207 = String To Byte Array(string=w323) -> (unsigned byte array=w321:u8[])
    "R45 ExB 1 command array" <- w321
    n208 = xnode "Read/Write Control"("FPGA VI Reference In"=w315, "error in"=w316, "ExB 1 PS set"=w321) -> ("error out"=w313:errorcluster)  [unwired: 1 out]
    "ExB 1 PS loop error" <- w313
    n209 = shared-variable ".\\local R45_2 shared var lib.lvlib\\ExB 1 PS loop error"(w313) -> ()  [unwired: 1 in, 1 out]
    n210 = node-c288() -> ()  [unwired: 1 in, 1 out]
  }
  n211 = node-c288(w7) -> ()  [unwired: 1 out]
  n212 = node-c288(w9) -> ()  [unwired: 1 out]
  n213 = node-c288(w11) -> ()  [unwired: 1 out]
  n214 = node-c288(w17) -> ()  [unwired: 1 out]
  n215 = node-c288(w5) -> ()  [unwired: 1 out]
  n216 = node-c288(w3) -> ()  [unwired: 1 out]
  n217 = node-c288(w19) -> ()  [unwired: 1 out]
  n218 = node-c288(w15) -> ()  [unwired: 1 out]
  n219 = node-c288(w13) -> ()  [unwired: 1 out]
